vi "Pump Module (Main).vi"(7 "Name of Parent Panel":string="Main.vi", 9 "New Center Coords":T1={"Horizontal"=470, "Vertical"=200}, 10 "Config":variant, 11 "Main UI Message Queue":refnum<queue>) -> ()   [LabVIEW 2018, in "Pump Module.lvlib"]
doc: "This Continuous Measurement sample project is based on the Queued Message Handler template.\n\nThe Event Handling Loop generates messages based on user interface actions.\n\nThe Message Handling Loop processes messages generated by the Event Handling Loop, or by other messages. There are also Acquisition and Logging message handling loop subVIs, and a chart updating loop."
uses:
  Pump Module.lvlib
  support/Message Queue/Message Cluster.ctl
  <vilib>/Utility/miscctls.llb/LVPoint32TypeDef.ctl
  controls/UI Data.ctl
  controls/UI State.ctl
  Pump Module State Cluster.ctl
  Pump Module Config Cluster.ctl
  Pump Module Settings Cluster.ctl
  Measure Instrument/PID 2 Output Enum.ctl
  Ismatec ISM 831C/Controls/Ismatech ISM831C Settings Cluster.ctl
  Ismatec 78001/Ismatec 4083.ctl
  Masterflex 7550-30/Controls/Settings Cluster.ctl
  VICI M50 Party Mode/Settings Cluster.ctl
  Tacmina QI/Tacmina QI DAQ Setting.ctl
  KNF Pump/Settings Cluster plus SIMDOS.ctl
  ASIA Pump/Pump Settings.ctl
  FLOM Pump/Settings Cluster.ctl
  SSI PR Class/SSI PR or LD Settings Cluster.ctl
  Masterflex 75211/Masterflex 75211 DAQ Setting.ctl
  Measure Instrument/State Enum.ctl
  Sequencing/Squence Update Cluster.ctl
  Pump Module Display.ctl
  support/Message Queue/Enqueue Message (Single).vi
  support/User Event - Stop/User Event - Stop.lvlib
  support/Support Library.lvlib
  support/Message Queue/Message Queue.lvlib
  Measure Instrument/Pump Module Engine.lvlib
  Masterflex 7550-30/Masterflex 7550-30.lvlib
  Ismatec ISM 831C/Ismatec ISM 831C.lvlib
  Measure Instrument/Feed Module Engine.lvlib
  Tacmina QI/Tacmina QI.lvlib
  KNF Pump/KNF SIMDOS.lvlib
  ASIA Pump.lvlib
  Sequencing/Sequencing Library.lvlib
  VICI M50 Party Mode/VICI M6 M50 Party Mode.lvlib
  Pump Settings Dialog.vi
  FLOM Pump/FLOM Pump.lvlib
  support/Command Log VIs/Command Logging.lvlib
  SSI PR Class/SSI PR or LD Pump.lvlib
  Masterflex 75211/Masterflex 75211.lvlib
  Ismatec 78001/Ismatec 4308.lvlib
  Report Generation/Report Generation.lvlib
panel:
  out "Calibration Enum":dbl
  in  "Settings Button":bool
  out "Original Width":u32
  out "Original Height":u32
  out "H/W":dbl
  out "Sequence Started":bool
  out "ScanCode":i16
  out "Log File path":path
  out "Status":string
  in  "Exit":bool
  out "Display Cluster":T2 {"Total ml" format="%#.1g"; "ml/min" format="%#_5g"; "PSIG" format="%#_5g"; "Pump %" format="%#_5g"}
  out "Ring":u16(ring)=2
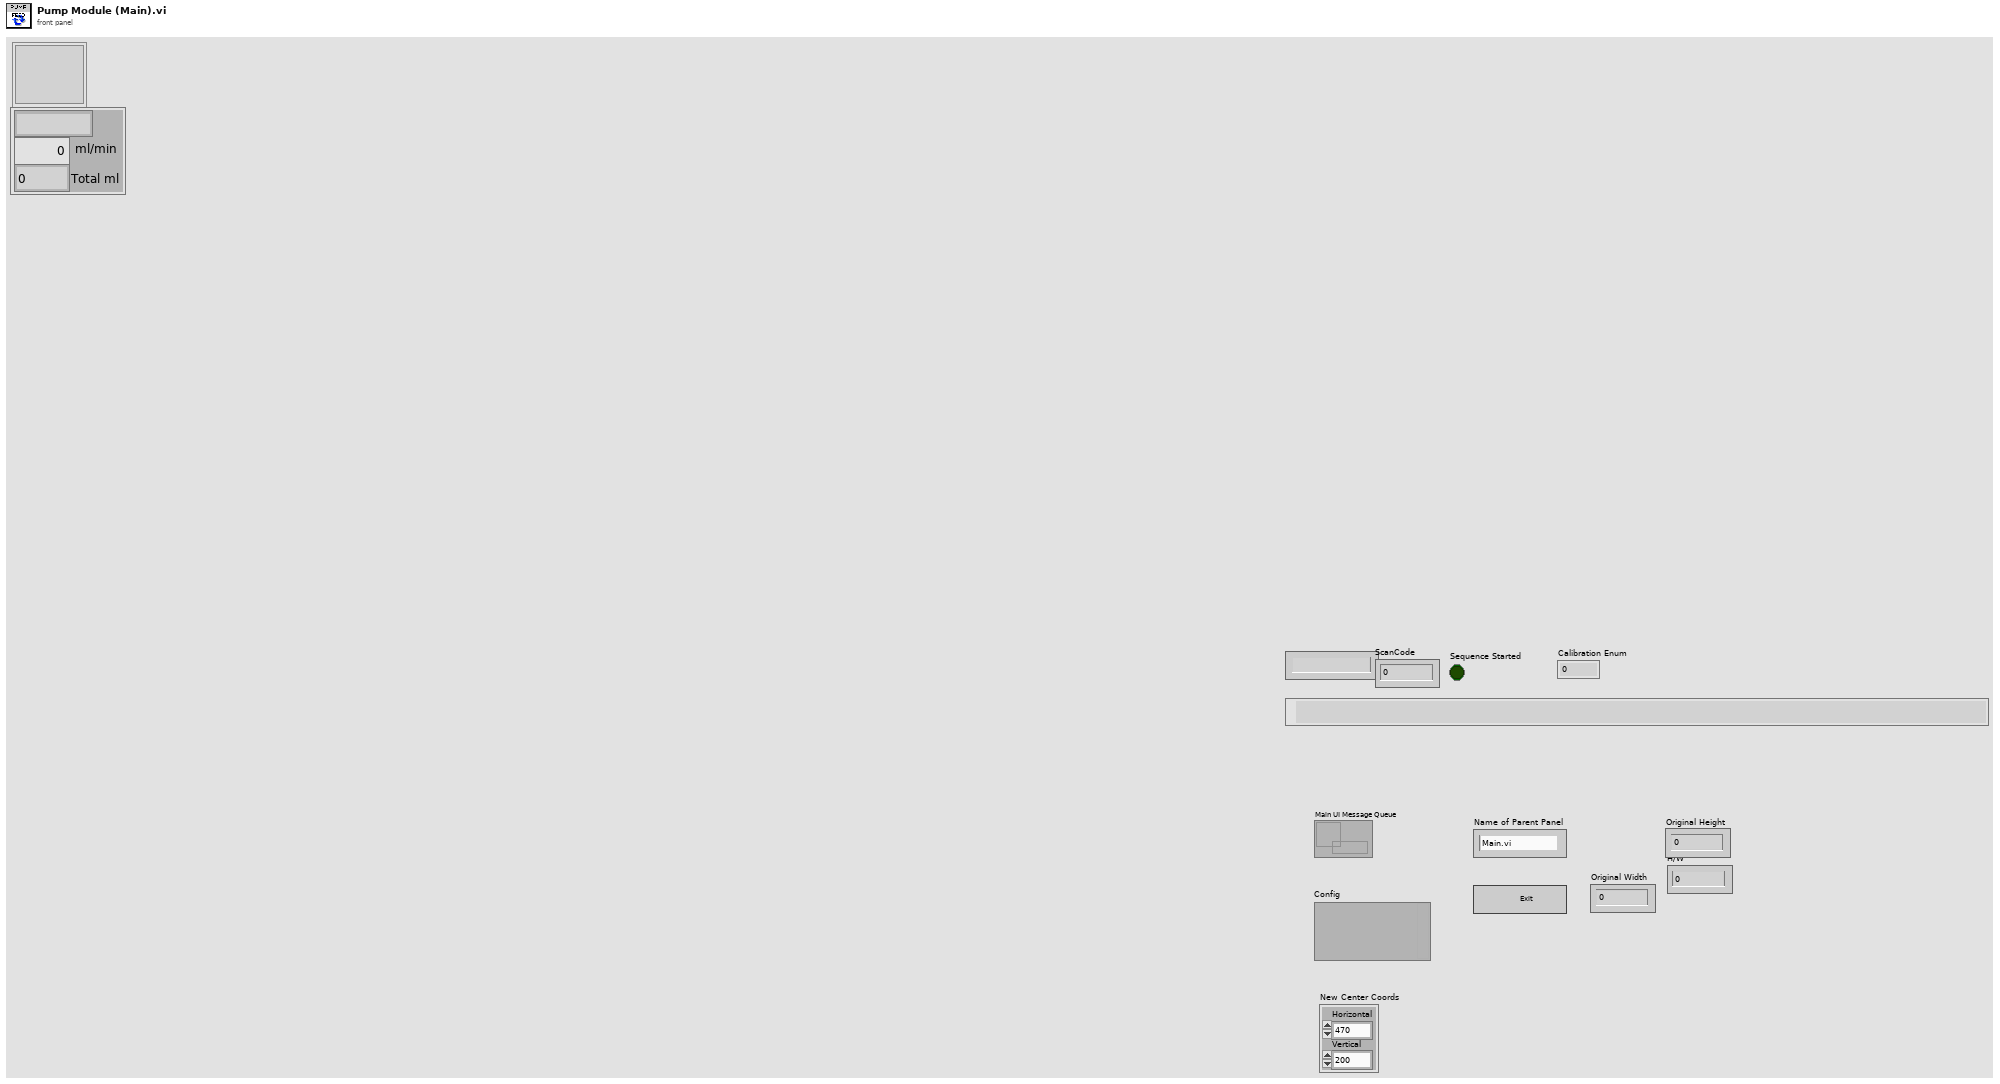
[diagram p1: front panel]
types:
  T1 = typedef "LVPoint32TypeDef.ctl" = cluster{"Horizontal":i32, "Vertical":i32}
  T2 = cluster{"User Name":string, "Pump %":dbl, "PSIG":dbl, "ml/min":dbl, "Total ml":dbl}
  T3 = typedef "Pump Module.lvlib/Pump Module Config Cluster.ctl" = cluster{"GUID":string, "Drop Coords":T1, "Process Name":string, "User name":string, "Queue Name":string, "Settings":T4, "Load Count":i32}
  T4 = typedef "Pump Module.lvlib/Pump Module Settings Cluster.ctl" = cluster{"Cycle Period":dbl, "Manual Entry":dbl, "Output Device":T5, "Ismatech":T6, "Ismatech 3 Channel Settings":T7, "Masterflex":T8, "VICI Settings":T9, "Tacmina Settings":T10, "KNF SIMDOS Settings":T11, "ASIA Pump C":T12, "FLOM Settings":T13, "SSI PR/LD Settings":T14, "SSI P40 Settings":T14, "Masterflex 75211 Settings":T15, "Pump Calibration File":path, "Calibration Slope":dbl, "Calibration Y Intercept":dbl, "Pump Cal Enum":u16, "Reset Totalizer":bool}
  T5 = typedef "PID 2 Output Enum.ctl" = enum16{"Default", "Ismatec ISM 4308", "Ismatec ISM 831C", "Masterflex 7550-30", "VICI M6", "VICI M50", "Tacmina QI", "KNF SIMDOS", "ASIA Type C", "FLOM UI-22-11", "SSI PR/LD", "SSI P40", "Masterflex 75211-70"}
  T6 = typedef "Ismatec ISM 831C.lvlib/Ismatech ISM831C Settings Cluster.ctl" = cluster{"VISA resource name":refnum<visa-resource-name>, "Simulated?":bool, "Pump Number":dbl, "Reverse?":bool}
  T7 = typedef "Ismatec 4308.lvlib/Ismatec 4083.ctl" = cluster{"VISA resource name":refnum<visa-resource-name>, "Pump Number":i16, "Channel Number":i16, "Simulated?":bool, "Reverse?":bool}
  T8 = typedef "Masterflex 7550-30.lvlib/Settings Cluster.ctl" = cluster{"VISA resource name":refnum<visa-resource-name>, "Simulated?":bool, "Pump Number":dbl, "Reverse?":bool}
  T9 = typedef "VICI M6 M50 Party Mode.lvlib/Settings Cluster.ctl" = cluster{"VISA resource name":refnum<visa-resource-name>, "Pump ID":string, "Pump Head Vol":dbl, "Reverse?":bool, "Simulated?":bool}
  T10 = typedef "Tacmina QI.lvlib/Tacmina QI DAQ Setting.ctl" = cluster{"Analog DAQ Task":refnum<k21>, "Digital DAQ Task":refnum<k21>}
  T11 = typedef "KNF SIMDOS.lvlib/Settings Cluster plus SIMDOS.ctl" = cluster{"VISA resource name":refnum<visa-resource-name>, "Simulated?":bool}
  T12 = typedef "ASIA Pump.lvlib/Pump Settings.ctl" = cluster{"ASIA Pump #":i32, "channel":i32, "Simulated":bool}
  T13 = typedef "FLOM Pump.lvlib/Settings Cluster.ctl" = cluster{"VISA resource name":refnum<visa-resource-name>, "Simulated?":bool, "Pump Number":dbl}
  T14 = typedef "SSI PR or LD Pump.lvlib/SSI PR or LD Settings Cluster.ctl" = cluster{"VISA resource name":refnum<visa-resource-name>, "Simulated?":bool}
  T15 = typedef "Masterflex 75211.lvlib/Masterflex 75211 DAQ Setting.ctl" = cluster{"Analog DAQ Task":refnum<k21>, "Digital DAQ Task":refnum<k21>}
  T16 = enum32{"Invalid", "Default", "Floating", "Floating/Auto-Hide", "Modal"}
  T17 = typedef "UI State.ctl" = enum16{"Idle", "Acquiring and Logging", "Waiting for Exit", "Waiting for Exit (Acq Stopped)", "Waiting for Exit (Log Stopped)", "Waiting for Stop", "Waiting for Stop (Acq Stopped)", "Waiting for Stop (Log Stopped)"}
  T18 = typedef "UI Data.ctl" = cluster{"Start Ref":refnum<vi>, "Trigger Ref":refnum<vi>, "Stop Ref":refnum<vi>, "Settings Ref":refnum<vi>, "Status Ref":refnum<vi>, "Exit Ref":refnum<vi>, "Data Ref":refnum<vi>}
  T19 = typedef "Pump Module.lvlib/Pump Module State Cluster.ctl" = cluster{"Pump Module Config":T3, "State":T20, "Start Time":timestamp, "Current Time":timestamp, "First Iteration":bool, "Data":cluster{"Pump Speed":dbl, "Totalized":dbl}, "Process Name":string, "Pump On?":bool}
  T20 = typedef "Feed Module.lvlib/Feed Module Engine.lvlib/State Enum.ctl" = enum16{"Measuring", "Idle", "Paused"}
  T21 = typedef "LVPointTypeDef.ctl" = cluster{"Horizontal":i16, "Vertical":i16}
  T22 = typedef "Pump Module.lvlib/All Message Queues.ctl" = cluster{"Engine":refnum<queue>, "Pump UI":refnum<queue>, "Pump Engine":refnum<queue>, "Pump Display":refnum<queue>}
  T23 = typedef "Pump Module.lvlib/Pump Module Display.ctl" = cluster{"Pump On?":enum16{"Off", "On", "Not Initialized"}, "Cycle Period":dbl, "Current Pump Speed":dbl, "Current Pump Pressure":dbl, "Current Pump Flow":dbl, "Totalized":dbl, "Output":T5}
  T24 = typedef "LVRectTypeDef.ctl" = cluster{"Left":i16, "Top":i16, "Right":i16, "Bottom":i16}
  T25 = cluster{"Shift":bool, "Ctrl":bool, "Alt":bool, "Cmd":bool, "Opt":bool}
  T26 = typedef "Sequencing Library.lvlib/Squence Update Cluster.ctl" = cluster{"Auto?":bool, "Manual Entry":dbl, "Setpoint":dbl}
  T27 = enum8{"Enabled", "Disabled", "Disabled and Grayed Out"}
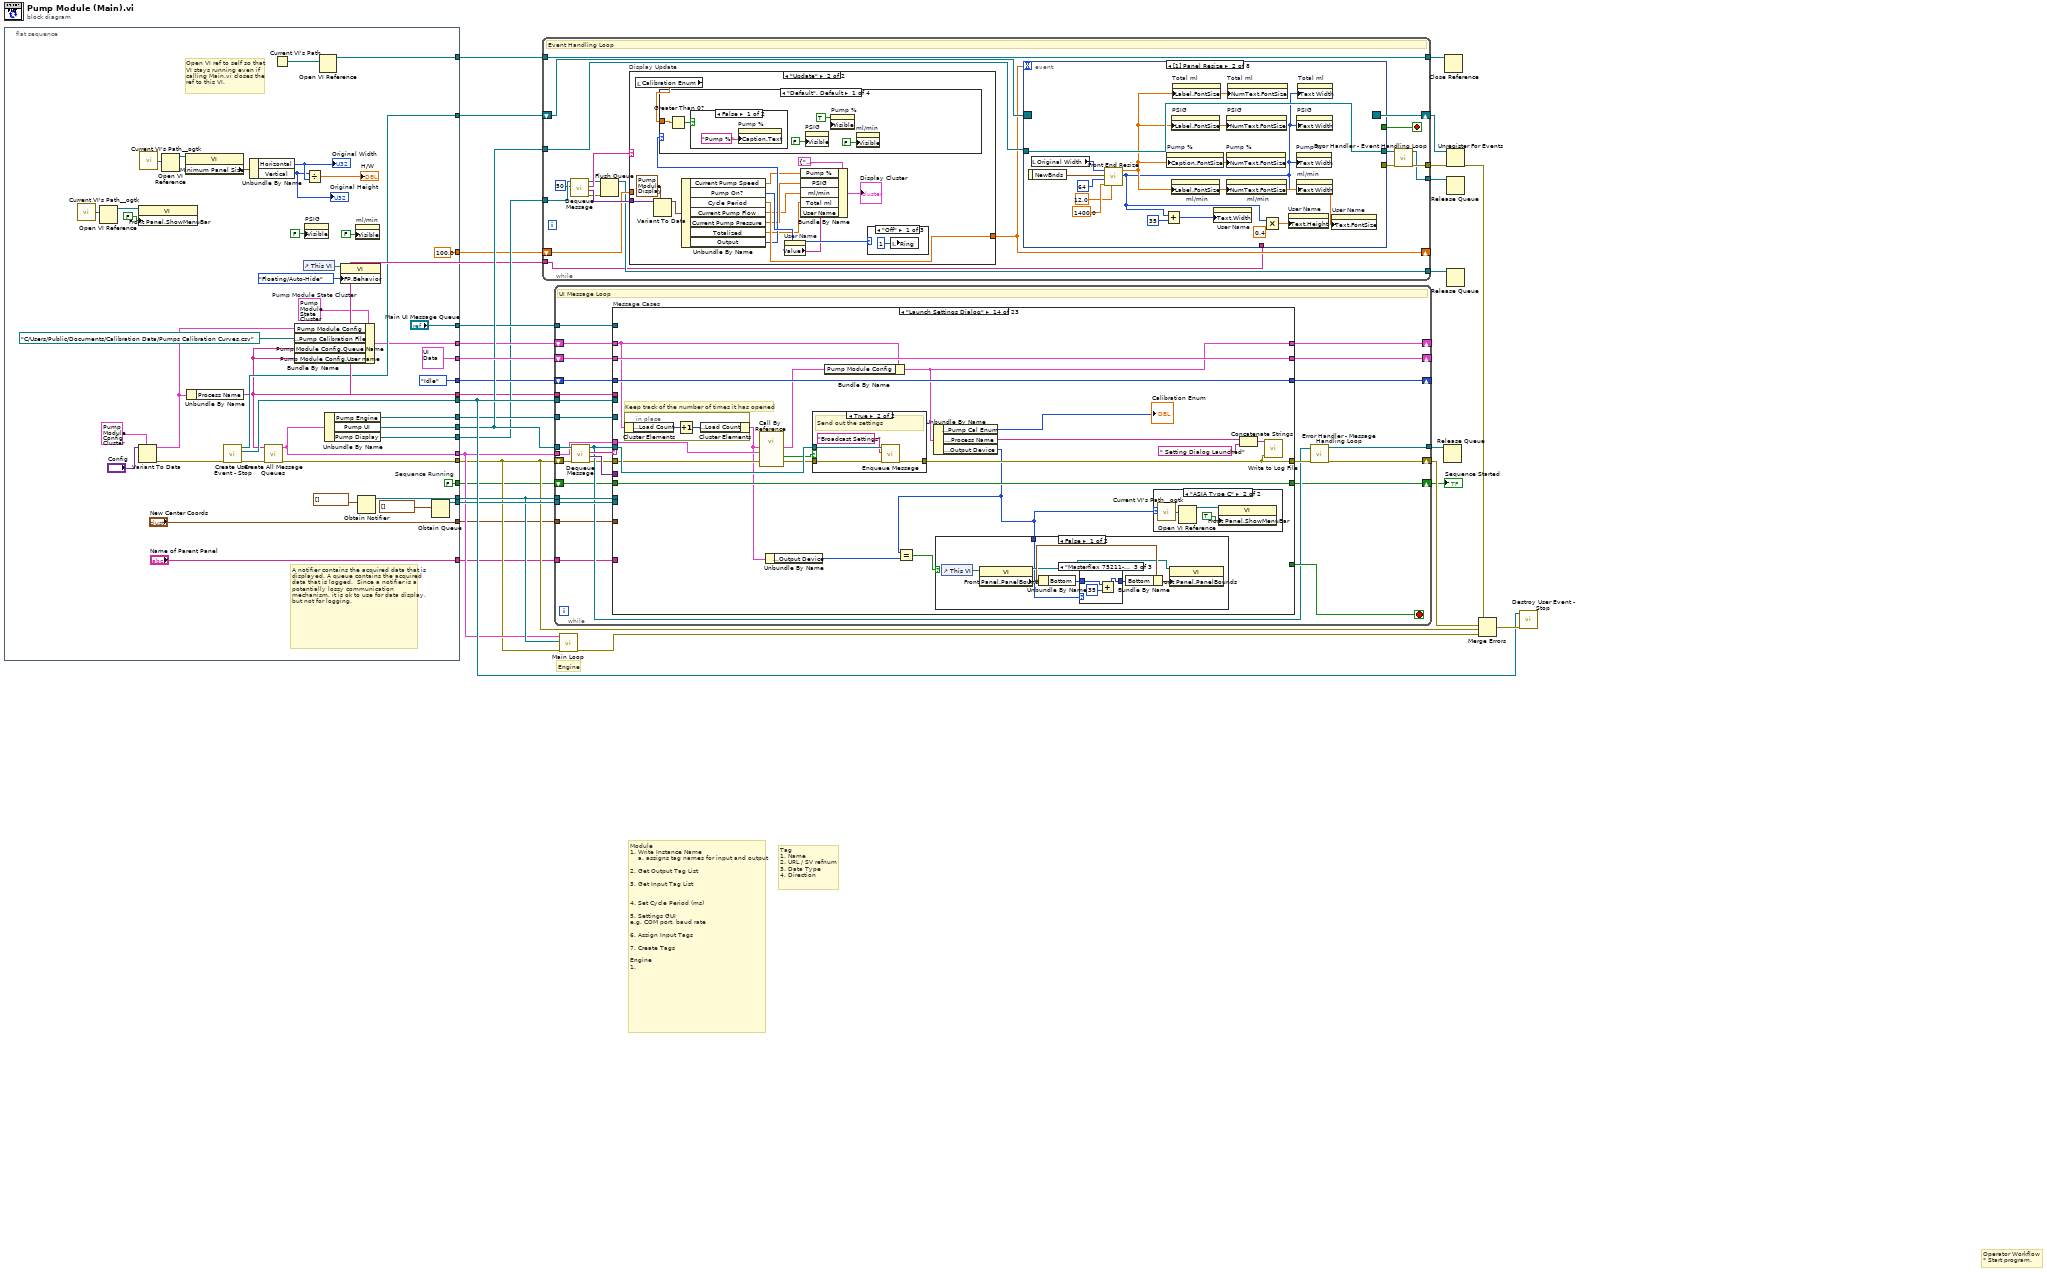
[diagram p0: block diagram]
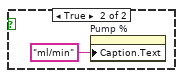
[diagram p3: hidden frame]
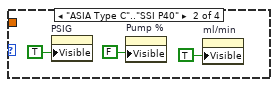
[diagram p4: hidden frame]
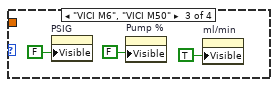
[diagram p5: hidden frame]
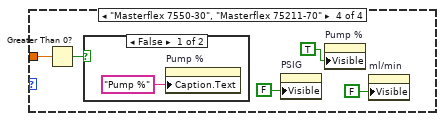
[diagram p6: hidden frame]
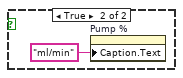
[diagram p7: hidden frame]
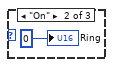
[diagram p8: hidden frame]
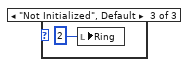
[diagram p9: hidden frame]
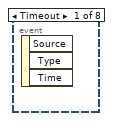
[diagram p10: hidden frame]
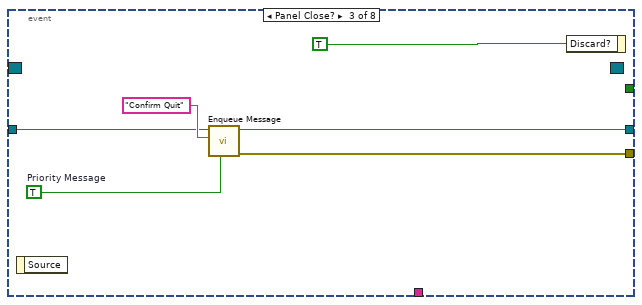
[diagram p11: hidden frame]
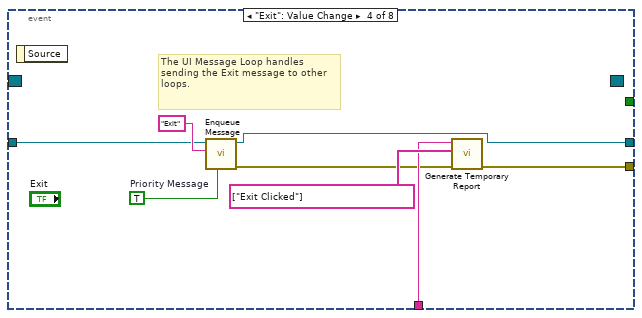
[diagram p12: hidden frame]
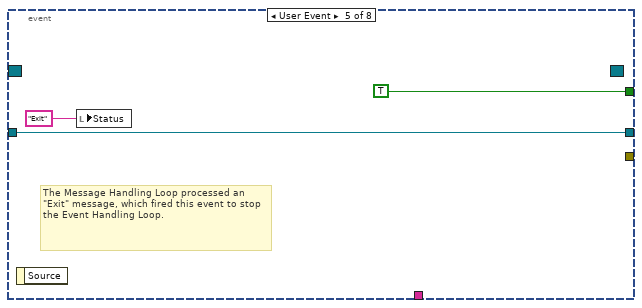
[diagram p13: hidden frame]
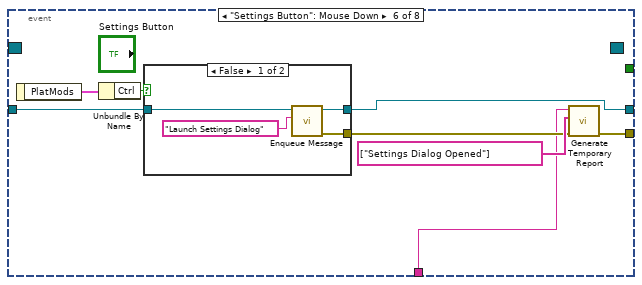
[diagram p14: hidden frame]
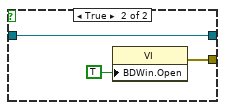
[diagram p15: hidden frame]
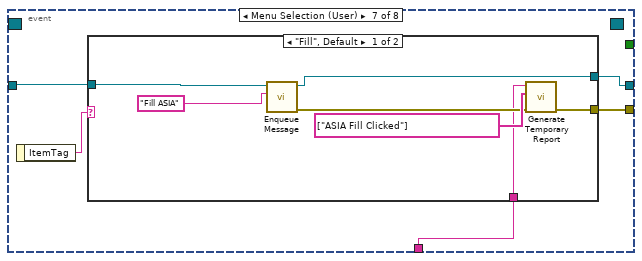
[diagram p16: hidden frame]
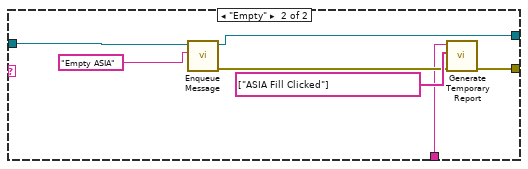
[diagram p17: hidden frame]
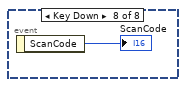
[diagram p18: hidden frame]
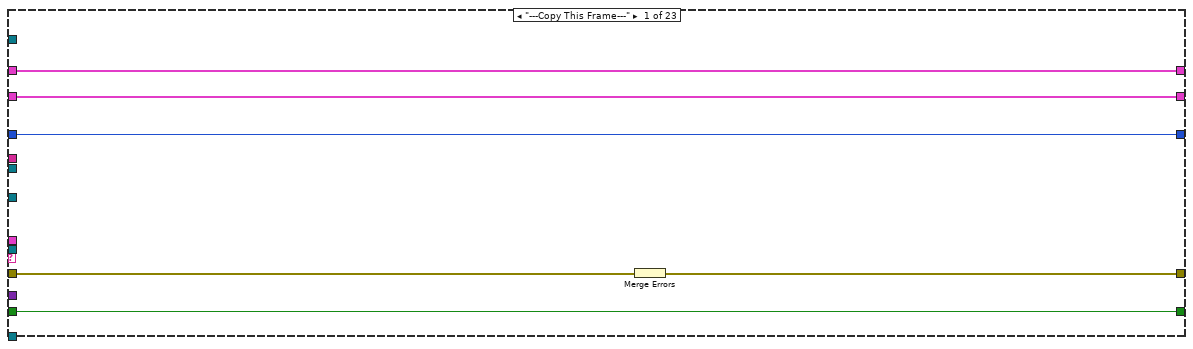
[diagram p19: hidden frame]
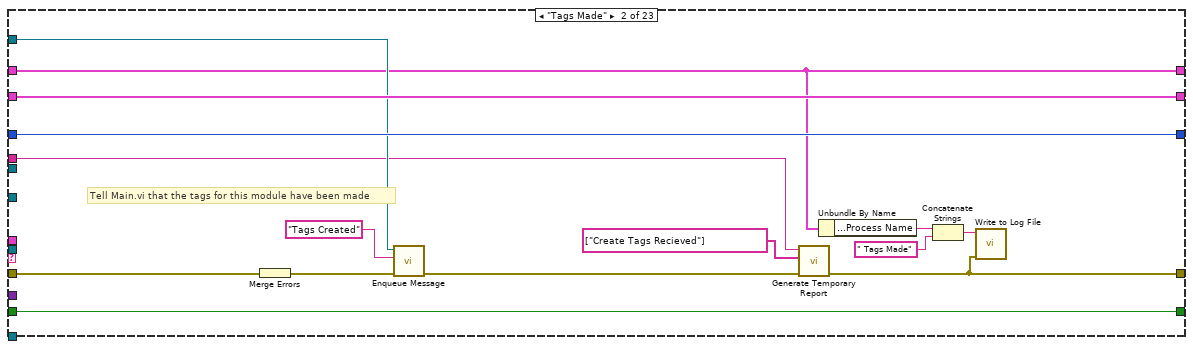
[diagram p20: hidden frame]
diagram:
  # "Engine"
  # "Operator Workflow\n* Start program."
  # "Module \n1. Write Instance Name\n    a. assigns tag names for input and output\n\n2. Get Output Tag List\n\n3. Get Input Tag List\n\n\n4. Set Cycle Period (ms)\n\n5. Settings GUI\ne.g. COM port, baud rate\n\n6. Assign Input Tags\n\n7. Create Tags\n\nEngine\n1."
  # "Tag\n1. Name\n2. URL / SV refnum\n3. Data Type\n4. Direction"
  n1 = flat-sequence {
    tunnel: [w72] -> w27
    tunnel: [w71] -> w26
    tunnel: [T18 {"Start Ref"=refnum, "Trigger Ref"=refnum, "Stop Ref"=refnum, "Settings Ref"=refnum, "Status Ref"=refnum, "Exit Ref"=refnum, "Data Ref"=refnum} ("Measurement UI Controls")] -> w23
    tunnel: [w69] -> w22
    tunnel: [UI_State."Idle" ("UI State")] -> w21
    tunnel: [w65] -> w20
    tunnel: [w64] -> w19
    tunnel: [w63] -> w17
    tunnel: [w62] -> w15
    tunnel: [w60] -> w14
    tunnel: ["Main UI Message Queue"] -> w13
    tunnel: [w55] -> w12
    tunnel: [w53] -> w11
    tunnel: [w52] -> w10
    tunnel: ["New Center Coords"] -> w9
    tunnel: ["Name of Parent Panel"] -> w8
    tunnel: [w49] -> w6
    tunnel: [100.0 ("Cycle Period")] -> w5
    tunnel: [w42] -> w1
    frame #0 {
      w49 = FALSE  # Sequence Running
      w56 = T19 {"Pump Module Config"={"GUID"="", "Drop Coords"={"Horizontal"=0, "Vertical"=0}, "Process Name"="", "User name"="", "Queue Name"="", "Settings"={"Cycle Period"=500.0, "Manual Entry"=0.0, "Output Device"=enum."VICI M6", "Ismatech"={"VISA resource name"="", "Simulated?"=TRUE, "Pump Number"=1.0, "Reverse?"=FALSE}, "Ismatech 3 Channel Settings"={"VISA resource name"="", "Pump Number"=1, "Channel Number"=0, "Simulated?"=TRUE, "Reverse?"=FALSE}, "Masterflex"={"VISA resource name"="", "Simulated?"=TRUE, "Pump Number"=1.0, "Reverse?"=FALSE}, "VICI Settings"={"VISA resource name"="", "Pump ID"="", "Pump Head Vol"=0.0, "Reverse?"=FALSE, "Simulated?"=TRUE}, "Tacmina Settings"={"Analog DAQ Task"="", "Digital DAQ Task"=""}, "KNF SIMDOS Settings"={"VISA resource name"="", "Simulated?"=TRUE}, "ASIA Pump C"={"ASIA Pump #"=0, "channel"=0, "Simulated"=FALSE}, "FLOM Settings"={"VISA resource name"="", "Simulated?"=TRUE, "Pump Number"=0.0}, "SSI PR/LD Settings"={"VISA resource name"="", "Simulated?"=FALSE}, "SSI P40 Settings"={"VISA resource name"="", "Simulated?"=FALSE}, "Masterflex 75211 Settings"={"Analog DAQ Task"="", "Digital DAQ Task"=""}, "Pump Calibration File"=path "", "Calibration Slope"=0.0, "Calibration Y Intercept"=0.0, "Pump Cal Enum"=0, "Reset Totalizer"=FALSE}, "Load Count"=0}, "State"=enum."Idle", "Start Time"=timestamp(0 s since 1904-01-01), "Current Time"=timestamp(0 s since 1904-01-01), "First Iteration"=FALSE, "Data"={"Pump Speed"=0.0, "Totalized"=0.0}, "Process Name"="", "Pump On?"=FALSE}  # Pump Module State Cluster
      # "Open VI ref to self so that\nVI stays running even if\ncalling Main.vi closes the\nref to this VI."
      # "A notifier contains the acquired data that is displayed. A queue contains the acquired data that is logged.  Since a notifier is a potentially lossy communication mechanism, it is ok to use for data display, but not for logging."
      n2 = call <userlib>:"Current VI's Path__ogtk.vi"() -> ("Current VI's Path (+ Relative)"=w33:path)  [unwired: 1 in]
      n3 = Open VI Reference(vi path=w33) -> (vi reference=w31:refnum<vi>)  [unwired: 5 in, 1 out]
      n4 = property class="VI"(reference=w31, "Front Panel.ShowMenuBar"=FALSE ("Front Panel Window:Show Menu Bar")) -> ()  [unwired: 1 in, 2 out]
      n5 = Variant To Data(type=T3 {"GUID"="", "Drop Coords"={"Horizontal"=0, "Vertical"=0}, "Process Name"="", "User name"="", "Queue Name"="", "Settings"={"Cycle Period"=500.0, "Manual Entry"=0.0, "Output Device"=enum."VICI M6", "Ismatech"={"VISA resource name"="", "Simulated?"=TRUE, "Pump Number"=1.0, "Reverse?"=FALSE}, "Ismatech 3 Channel Settings"={"VISA resource name"="", "Pump Number"=1, "Channel Number"=0, "Simulated?"=TRUE, "Reverse?"=FALSE}, "Masterflex"={"VISA resource name"="", "Simulated?"=TRUE, "Pump Number"=1.0, "Reverse?"=FALSE}, "VICI Settings"={"VISA resource name"="", "Pump ID"="", "Pump Head Vol"=0.0, "Reverse?"=FALSE, "Simulated?"=TRUE}, "Tacmina Settings"={"Analog DAQ Task"="", "Digital DAQ Task"=""}, "KNF SIMDOS Settings"={"VISA resource name"="", "Simulated?"=TRUE}, "ASIA Pump C"={"ASIA Pump #"=0, "channel"=0, "Simulated"=FALSE}, "FLOM Settings"={"VISA resource name"="", "Simulated?"=TRUE, "Pump Number"=0.0}, "SSI PR/LD Settings"={"VISA resource name"="", "Simulated?"=FALSE}, "SSI P40 Settings"={"VISA resource name"="", "Simulated?"=FALSE}, "Masterflex 75211 Settings"={"Analog DAQ Task"="", "Digital DAQ Task"=""}, "Pump Calibration File"=path "", "Calibration Slope"=0.0, "Calibration Y Intercept"=0.0, "Pump Cal Enum"=0, "Reset Totalizer"=FALSE}, "Load Count"=0} ("Feed Module Config"), Variant="Config") -> (data=w58:T3, error out=w59:errorcluster)  [unwired: 1 in]
      n6 = call <userlib>:"Current VI's Path__ogtk.vi"() -> ("Current VI's Path (+ Relative)"=w38:path)  [unwired: 1 in]
      n7 = Open VI Reference(vi path=w38) -> (vi reference=w37:refnum<vi>)  [unwired: 5 in, 1 out]
      n8 = property class="VI"(reference=w37) -> ("Minimum Panel Size"=w36:T21)  [unwired: 1 in, 2 out]
      n9 = Unbundle By Name(w58) -> ("Process Name"=w42:string)
      n10 = call "Create User Event - Stop.vi"("error in (no error)"=w59) -> ("error out"=w54:errorcluster, "User Event - Stop"=w71:refnum<user-event>, "Stop Event Registration Refnum"=w72:refnum<event-registration>)  [unwired: 8 in]
      n11 = Unbundle By Name(w36) -> ("Horizontal"=w35:i16, "Vertical"=w34:i16)
      "Original Width" <- w35
      "Original Height" <- w34
      n12 = call "Create All Message Queues.vi"("error in (no error)"=w54, "Process Name"=w42) -> ("error out"=w52:errorcluster, "Message Queues"=w53:T22)  [unwired: 8 in]
      n13 = Current VI's Path() -> (path=w61:path)
      n14 = Bundle By Name(cluster=w56, "Pump Module Config"=w58, "Pump Module Config.Settings.Pump Calibration File"=path "C:/Users/Public/Documents/Calibration Data/Pumps Calibration Curves.csv", "Pump Module Config.Queue Name"=w42, "Pump Module Config.User name"=w42) -> (w60:T19)
      n15 = control-ref of="This VI"() -> (w44:refnum<vi>)
      n16 = property on="PSIG" class="DigNum (strict)"("Visible"=FALSE) -> ()  [unwired: 2 in, 2 out]
      n17 = Divide(x=w34, y=w35) -> (x/y=→"H/W":dbl)
      n18 = Open VI Reference(vi path=w61) -> (vi reference=w62:refnum<vi>)  [unwired: 5 in, 1 out]
      n19 = Unbundle By Name(w53) -> ("Pump Engine"=w65:refnum<queue>, "Pump UI"=w69:refnum<queue>, "Pump Display"=w55:refnum<queue>)
      n20 = property class="VI"(reference=w44, "FP.Behavior"=T16."Floating/Auto-Hide" ("Front Panel Window:Behavior")) -> ()  [unwired: 1 in, 2 out]
      n21 = property on="ml/min" class="DigNum (strict)"("Visible"=FALSE) -> ()  [unwired: 2 in, 2 out]
      n22 = Obtain Notifier(notification data type=waveform(dbl)[] []) -> (notifier out=w63:refnum<notifier>)  [unwired: 3 in, 2 out]
      n23 = Obtain Queue(element data type=waveform(dbl)[] []) -> (queue out=w64:refnum<queue>)  [unwired: 4 in, 2 out]
    }
  }
  n24 = while {
    tunnel: w22 -> [w85]
    tunnel: [w87] -> w29
    shift-right: [w86] -> w24
    shift-left: w27 -> [w91]
    tunnel: [w84] -> w16
    tunnel: w15 -> [w84]
    tunnel: w12 -> [w83]
    shift-right: [w80] -> _
    shift-left: w5 -> [w79]
    tunnel: [w75] -> w4
    tunnel: [w74] -> w3
    tunnel: w1 -> [w73]
    stop <- w90 stop-if-true
    # "Event Handling Loop"
    n25 = call "Dequeue Message.vi"("timeout in ms (-1)"=50, "Message Queue"=w83) -> ("error out"=w76:errorcluster, "Message Data"=w81:variant, "Message"=w82:string, "dup Message Queue"=w77:refnum<queue>)  [unwired: 6 in]
    n26 = Flush Queue(queue=w77, error in (no error)=w76) -> (queue out=w74:refnum<queue>)  [unwired: 2 out]
    n27 = case "Display Update" shown="\"Update\"" w82 {
      tunnel: w81 -> [_ w106]
      tunnel: [w92 w103] -> w80
      tunnel: w79 -> [w92 _]
      frame "False", Default {
      }
      frame "Update" {
        n28 = local read "Calibration Enum"() -> (w95:dbl)
        n29 = Variant To Data(type=T23 {"Pump On?"=enum."Off", "Cycle Period"=500.0, "Current Pump Speed"=0.0, "Current Pump Pressure"=0.0, "Current Pump Flow"=0.0, "Totalized"=0.0, "Output"=enum."Default"} ("FM Display"), Variant=w106) -> (data=w105:T23)  [unwired: 1 in, 1 out]
        n30 = Unbundle By Name(w105) -> ("Current Pump Speed"=w99:dbl, "Pump On?"=w104:enum16{"Off", "On", "Not Initialized"}, "Cycle Period"=w103:dbl, "Current Pump Flow"=w98:dbl, "Current Pump Pressure"=w100:dbl, "Totalized"=w96:dbl, "Output"=w101:T5)
        n31 = case shown="\"Default\", Default" w101 {
          tunnel: w95 -> [w107 _ _ w120]
          frame "Default", Default {
            n32 = Greater Than 0?(x=w107) -> (x > 0?=w108:bool)
            n33 = case shown="False" w108 {
              frame False {
                n34 = property on="Pump %" class="DigNum (strict)"("Caption.Text"="Pump %" ("Label.Text")) -> ()  [unwired: 2 in, 2 out]
              }
              frame True {
                n35 = property on="Pump %" class="DigNum (strict)"("Caption.Text"="ml/min" ("Label.Text")) -> ()  [unwired: 2 in, 2 out]
              }
            }
            n36 = property on="PSIG" class="DigNum (strict)"("Visible"=FALSE) -> ()  [unwired: 2 in, 2 out]
            n37 = property on="Pump %" class="DigNum (strict)"("Visible"=TRUE) -> ()  [unwired: 2 in, 2 out]
            n38 = property on="ml/min" class="DigNum (strict)"("Visible"=FALSE) -> ()  [unwired: 2 in, 2 out]
          }
          frame "ASIA Type C".."SSI P40" {
            n39 = property on="PSIG" class="DigNum (strict)"("Visible"=TRUE) -> ()  [unwired: 2 in, 2 out]
            n40 = property on="Pump %" class="DigNum (strict)"("Visible"=FALSE) -> ()  [unwired: 2 in, 2 out]
            n41 = property on="ml/min" class="DigNum (strict)"("Visible"=TRUE) -> ()  [unwired: 2 in, 2 out]
          }
          frame "VICI M6", "VICI M50" {
            n42 = property on="PSIG" class="DigNum (strict)"("Visible"=FALSE) -> ()  [unwired: 2 in, 2 out]
            n43 = property on="Pump %" class="DigNum (strict)"("Visible"=FALSE) -> ()  [unwired: 2 in, 2 out]
            n44 = property on="ml/min" class="DigNum (strict)"("Visible"=TRUE) -> ()  [unwired: 2 in, 2 out]
          }
          frame "Masterflex 7550-30", "Masterflex 75211-70" {
            n45 = Greater Than 0?(x=w120) -> (x > 0?=w121:bool)
            n46 = case shown="False" w121 {
              frame False {
                n47 = property on="Pump %" class="DigNum (strict)"("Caption.Text"="Pump %" ("Label.Text")) -> ()  [unwired: 2 in, 2 out]
              }
              frame True {
                n48 = property on="Pump %" class="DigNum (strict)"("Caption.Text"="ml/min" ("Label.Text")) -> ()  [unwired: 2 in, 2 out]
              }
            }
            n49 = property on="PSIG" class="DigNum (strict)"("Visible"=FALSE) -> ()  [unwired: 2 in, 2 out]
            n50 = property on="Pump %" class="DigNum (strict)"("Visible"=TRUE) -> ()  [unwired: 2 in, 2 out]
            n51 = property on="ml/min" class="DigNum (strict)"("Visible"=FALSE) -> ()  [unwired: 2 in, 2 out]
          }
        }
        n52 = property on="User Name" class="Str"() -> ("Value"=w93:string)  [unwired: 2 in, 2 out]
        n53 = Bundle By Name(cluster=T2 {"User Name"="", "Pump %"=0.0, "PSIG"=0.0, "ml/min"=0.0, "Total ml"=0.0} ("Display Cluster"), "Pump %"=w99, "PSIG"=w100, "ml/min"=w98, "Total ml"=w96, "User Name"=w93) -> (→"Display Cluster":T2)
        n54 = case shown="\"Off\"" w104 {
          frame "Off" {
            n55 = local write "Ring"(u16 1 ("Ring")) -> ()
          }
          frame "On" {
            "Ring" <- u16 0 ("Ring")
          }
          frame "Not Initialized", Default {
            n56 = local write "Ring"(u16 2 ("Ring")) -> ()
          }
        }
      }
    }
    n57 = event shown="[1] Panel Resize" {
      selector: w91 -> [_ _ _ _ _ _ _ _]
      dyn-events: [_ _ _ _ _ _ _ _] -> w86
      timeout: w80 -> [_ _ _ _ _ _ _ _]
      tunnel: [_ _ _ _ TRUE ("Discard?") _ _ _] -> w90
      tunnel: w85 -> [_ w141 w144 w153 w156 w165 w178 _]
      tunnel: [_ _ w142 w148 _ w160 w176 _] -> w88
      tunnel: [_ w141 w143 w152 w156 w166 w175 _] -> w89
      tunnel: w73 -> [_ _ _ w150 _ w159 w174 _]
      event Timeout {
        n58 = event-data() -> ()  [unwired: 1 in, 3 out]
      }
      event Panel Resize {
        n59 = event-data() -> ("NewBnds"=w136:T24)  [unwired: 1 in]
        n60 = local read "Original Width"() -> (w137:u32)
        n61 = call "Front End Resize.vi"("Starting Font"=12.0, "Area to Font Division"=1400.0, "Original Text Box Width"=64, "NewBnds"=w136, "Original Panel Width"=w137) -> ("New Text Box Width"=w130:u64, "New Font Size"=w135:dbl)  [unwired: 5 in]
        n62 = Add(x=w130, y=u64 35) -> (x+y=w131:u64)
        n63 = property on="Pump %" class="DigNum (strict)"("Caption.FontSize"=w135) -> ()  [unwired: 2 in, 2 out]
        n64 = property on="PSIG" class="DigNum (strict)"("Label.FontSize"=w135) -> ()  [unwired: 2 in, 2 out]
        n65 = property on="ml/min" class="DigNum (strict)"("Label.FontSize"=w135) -> ()  [unwired: 2 in, 2 out]
        n66 = property on="Total ml" class="DigNum (strict)"("Label.FontSize"=w135) -> ()  [unwired: 2 in, 2 out]
        n67 = property on="User Name" class="Str"("Text.Width"=w131) -> ()  [unwired: 2 in, 2 out]
        n68 = property on="Pump %" class="DigNum (strict)"("NumText.FontSize"=w135) -> ()  [unwired: 2 in, 2 out]
        n69 = property on="PSIG" class="DigNum (strict)"("NumText.FontSize"=w135) -> ()  [unwired: 2 in, 2 out]
        n70 = property on="ml/min" class="DigNum (strict)"("NumText.FontSize"=w135) -> ()  [unwired: 2 in, 2 out]
        n71 = property on="Total ml" class="DigNum (strict)"("NumText.FontSize"=w135) -> ()  [unwired: 2 in, 2 out]
        n72 = Multiply(x=w130, y=0.4) -> (x*y=w134:dbl)
        n73 = property on="User Name" class="Str"("Text.Height"=w134) -> ()  [unwired: 2 in, 2 out]
        n74 = property on="Pump %" class="DigNum (strict)"("Text Width"=w130) -> ()  [unwired: 2 in, 2 out]
        n75 = property on="PSIG" class="DigNum (strict)"("Text Width"=w130) -> ()  [unwired: 2 in, 2 out]
        n76 = property on="ml/min" class="DigNum (strict)"("Text Width"=w130) -> ()  [unwired: 2 in, 2 out]
        n77 = property on="Total ml" class="DigNum (strict)"("Text Width"=w130) -> ()  [unwired: 2 in, 2 out]
        n78 = property on="User Name" class="Str"("Text.FontSize"=w135) -> ()  [unwired: 2 in, 2 out]
      }
      event Panel Close? {
        w145 = TRUE  # Priority Message
        n79 = event-data() -> ()  [unwired: 1 in, 1 out]
        n80 = call-poly "Enqueue Message.vi"("Priority Message? (F)"=w145, "Message"="Confirm Quit", "Message Queue"=w144) -> ("error out"=w142:errorcluster, "dup Message Queue"=w143:refnum<queue>)  [unwired: 7 in]
        n81 = event-data("Discard?"=TRUE) -> ()  [unwired: 1 in, 1 out]
      }
      event "Exit": Value Change {
        w154 = TRUE  # Priority Message
        # "The UI Message Loop handles sending the Exit message to other loops."
        n82 = event-data() -> ()  [unwired: 1 in, 1 out]
        n83 = call-poly "Enqueue Message.vi"("Priority Message? (F)"=w154, "Message"="Exit", "Message Queue"=w153) -> ("error out"=w149:errorcluster, "dup Message Queue"=w152:refnum<queue>)  [unwired: 7 in]
        n84 = call "Generate Temporary Report.vi"("error in (no error)"=w149, "Line of Events"=string[] ["Exit Clicked"], "Module Name"=w150) -> ("error out"=w148:errorcluster)  [unwired: 8 in]
      }
      event User Event {
        # "The Message Handling Loop processed an \"Exit\" message, which fired this event to stop the Event Handling Loop."
        n85 = event-data() -> ()  [unwired: 1 in, 1 out]
        n86 = local write "Status"("Exit" ("Exit String")) -> ()
      }
      event "Settings Button": Mouse Down {
        n87 = event-data() -> ("PlatMods"=w164:T25)  [unwired: 1 in]
        n88 = Unbundle By Name(w164) -> ("Ctrl"=w163:bool)
        n89 = case shown="False" w163 {
          tunnel: [w170 w171] -> w161
          tunnel: [w169 w172] -> w166
          tunnel: w165 -> [w168 w172]
          frame False {
            n90 = call-poly "Enqueue Message.vi"("Message"="Launch Settings Dialog", "Message Queue"=w168) -> ("error out"=w170:errorcluster, "dup Message Queue"=w169:refnum<queue>)  [unwired: 8 in]
          }
          frame True {
            n91 = property class="VI"("BDWin.Open"=TRUE ("Block Diagram Window:Open")) -> (error out=w171:errorcluster)  [unwired: 2 in, 1 out]
          }
        }
        n92 = call "Generate Temporary Report.vi"("error in (no error)"=w161, "Line of Events"=string[] ["Settings Dialog Opened"], "Module Name"=w159) -> ("error out"=w160:errorcluster)  [unwired: 8 in]
      }
      event Menu Selection (User) {
        n93 = event-data() -> ("ItemTag"=w177:string)  [unwired: 1 in]
        n94 = case shown="\"Fill\", Default" w177 {
          tunnel: w178 -> [w184 w191]
          tunnel: [w182 w189] -> w176
          tunnel: [w180 w187] -> w175
          tunnel: w174 -> [w179 w186]
          frame "Fill", Default {
            n95 = call-poly "Enqueue Message.vi"("Message"="Fill ASIA", "Message Queue"=w184) -> ("error out"=w181:errorcluster, "dup Message Queue"=w180:refnum<queue>)  [unwired: 8 in]
            n96 = call "Generate Temporary Report.vi"("error in (no error)"=w181, "Line of Events"=string[] ["ASIA Fill Clicked"], "Module Name"=w179) -> ("error out"=w182:errorcluster)  [unwired: 8 in]
          }
          frame "Empty" {
            n97 = call-poly "Enqueue Message.vi"("Message"="Empty ASIA", "Message Queue"=w191) -> ("error out"=w188:errorcluster, "dup Message Queue"=w187:refnum<queue>)  [unwired: 8 in]
            n98 = call "Generate Temporary Report.vi"("error in (no error)"=w188, "Line of Events"=string[] ["ASIA Fill Clicked"], "Module Name"=w186) -> ("error out"=w189:errorcluster)  [unwired: 8 in]
          }
        }
      }
      event Key Down {
        n99 = event-data() -> ("ScanCode"=→"ScanCode":i16)  [unwired: 1 in]
      }
    }
    n100 = call "Error Handler - Event Handling Loop.vi"("error in (no error)"=w88, "Message Queue"=w89) -> ("dup error in"=w87:errorcluster, "dup Message Queue"=w75:refnum<queue>)  [unwired: 8 in]
  }
  n101 = while {
    tunnel: w22 -> [w215]
    tunnel: w26 -> [w219]
    shift-right: [w209] -> w30
    shift-left: w10 -> [w218]
    shift-right: [w202] -> _
    shift-left: w14 -> [w195]
    shift-right: [w213] -> _
    shift-left: w23 -> [w214]
    tunnel: w17 -> [w212]
    tunnel: w19 -> [w211]
    shift-right: [w206] -> _
    shift-left: w21 -> [w207]
    tunnel: w20 -> [w205]
    tunnel: w13 -> [w203]
    tunnel: w11 -> [w201]
    tunnel: w1 -> [w200]
    tunnel: w9 -> [w199]
    tunnel: w8 -> [w198]
    shift-right: [w197] -> w7
    shift-left: w6 -> [w196]
    tunnel: [w194] -> w2
    stop <- w220 stop-if-true
    # "UI Message Loop"
    n102 = call "Dequeue Message.vi"("error in (no error)"=w218, "Message Queue"=w215) -> ("error out"=w204:errorcluster, "Message Data"=w216:variant, "Message"=w217:string, "dup Message Queue"=w208:refnum<queue>)  [unwired: 6 in]
    n103 = case "Message Cases" shown="\"Launch Settings Dialog\"" w217 {
      selector: w217 -> [_ _ _ _ _ _ _ _ _ _ _ _ _ _ _ _ _ _ _ _ _ w754 w770]
      tunnel: w208 -> [_ _ w248 _ w324 _ w360 _ w427 w442 w472 _ w510 w534 w572 w608 w647 _ _ w711 _ _ _]
      tunnel: w204 -> [w226 w241 w249 w283 w323 w345 w359 w392 w408 w446 w476 w492 w505 w533 w573 w606 w646 w671 w684 w713 w747 w758 _]
      tunnel: [w225 w227 w244 w275 w319 w343 w357 w393 w399 w431 w448 w492 w493 w524 w567 w595 w634 w666 w686 w702 w748 w757 w769] -> w210
      tunnel: [_ _ _ _ _ _ _ _ _ _ TRUE _ _ _ _ _ _ _ _ _ _ _ _] -> w220
      tunnel: w216 -> [_ _ _ _ w325 w342 _ w395 _ w445 w460 _ _ _ _ _ _ _ _ _ w746 _ _]
      tunnel: w219 -> [_ _ _ _ _ _ _ _ _ _ w475 _ _ _ _ _ _ _ _ _ _ _ _]
      tunnel: w195 -> [w222 w232 w243 w288 w317 w352 w356 w390 w406 w433 w453 w483 w498 w523 w568 w599 w642 w672 w685 w715 w737 w756 w775]
      tunnel: w214 -> [w224 w240 w252 w301 w326 w354 w362 w397 w424 w447 w473 w491 w506 w536 w576 w603 w643 w677 w695 w731 w743 w762 w780]
      tunnel: [w224 w240 w252 w301 w326 w354 w362 w397 w424 w447 w473 w490 w506 w536 w576 w603 w643 w677 w695 w731 w743 w762 w780] -> w213
      tunnel: w212 -> [_ _ _ _ _ _ _ _ _ _ w471 _ _ _ _ _ _ _ _ _ _ _ _]
      tunnel: w211 -> [_ _ _ _ _ _ _ _ _ _ w467 _ _ _ _ _ _ _ _ _ _ _ _]
      tunnel: w207 -> [w223 w239 w251 w300 w327 w353 w361 w391 w413 w437 _ _ _ w535 w575 _ _ _ _ w720 w738 w760 w779]
      tunnel: [w223 w239 w250 w300 w327 w353 w358 w391 w414 w437 UI_State."Idle" ("UI State") UI_State."Idle" ("UI State") UI_State."Idle" ("UI State") w535 w574 UI_State."Acquiring and Logging" ("UI State") UI_State."Acquiring and Logging" ("UI State") UI_State."Acquiring and Logging" ("UI State") UI_State."Acquiring and Logging" ("UI State") w721 w738 w760 w779] -> w206
      tunnel: w205 -> [_ _ _ w292 _ _ _ _ w412 _ w459 _ _ _ _ _ _ w675 w693 w719 _ w759 _]
      tunnel: w203 -> [_ w236 _ w298 _ _ _ _ _ _ w461 _ _ _ _ _ _ _ _ _ _ _ _]
      tunnel: [w222 w232 w243 w288 w316 w352 w356 w390 w403 w433 w453 w483 w498 w525 w568 w598 w633 w672 w685 w706 w737 w756 w775] -> w202
      tunnel: w201 -> [_ _ _ w296 _ _ _ _ _ _ _ _ _ w532 _ _ _ _ _ _ _ _ _]
      tunnel: w200 -> [_ w229 _ _ _ _ _ _ _ _ _ _ w501 _ _ _ _ _ _ _ _ _ _]
      tunnel: w199 -> [_ _ _ _ _ _ _ _ _ _ _ _ w503 _ _ _ _ _ _ _ _ _ _]
      tunnel: w198 -> [_ _ _ _ _ _ _ _ _ _ _ _ w502 _ _ _ _ _ _ _ _ _ _]
      tunnel: [w221 w231 w242 w286 w315 w351 w355 w389 w402 w430 w452 w482 w497 w522 w566 w597 w640 w670 w683 w705 w736 w761 w768] -> w197
      tunnel: w196 -> [w221 w231 w242 w286 w315 w351 w355 w389 w402 w430 w452 w482 w497 w522 w566 w597 w638 w670 w683 w705 w736 w761 w768]
      frame "---Copy This Frame---" {
        # "Duplicate this frame when creating new messages.  Change this comment in the duplicated frame to describe this message."
        n104 = Merge Errors(w226) -> (w225:errorcluster)
      }
      frame "Tags Made" {
        # "Tell Main.vi that the tags for this module have been made"
        # "Duplicate this frame when creating new messages.  Change this comment in the duplicated frame to describe this message."
        n105 = Merge Errors(w241) -> (w237:errorcluster)
        n106 = call-poly "Enqueue Message.vi"("error in (no error)"=w237, "Message"="Tags Created", "Message Queue"=w236) -> ("error out"=w228:errorcluster)  [unwired: 7 in, 1 out]
        n107 = call "Generate Temporary Report.vi"("error in (no error)"=w228, "Line of Events"=string[] ["Create Tags Recieved"], "Module Name"=w229) -> ("error out"=w227:errorcluster)  [unwired: 8 in]
        n108 = Unbundle By Name(w232) -> ("Pump Module Config.Process Name"=w235:string)
        n109 = Concatenate Strings(w235, " Tags Made" ("text")) -> (w233:string)
        n110 = call "Write to Log File.vi"("error in"=w227, "text"=w233) -> ()  [unwired: 9 in, 1 out]
      }
      frame "Acquisition Stopped" {
        # "Logic for determining what action to take when the acquisition has stopped."
        n111 = case shown="\"Waiting for Stop (Log Stopped)\"" w251 {
          selector: w251 -> [w254 _ _ _ _]
          tunnel: [w254 UI_State."Waiting for Exit (Acq Stopped)" ("UI State") UI_State."Waiting for Stop (Acq Stopped)" ("UI State") UI_State."Idle" ("UI State") UI_State."Idle" ("UI State")] -> w250
          tunnel: w249 -> [w253 w255 w257 w263 w269]
          tunnel: [w253 w255 w257 w262 w268] -> w244
          tunnel: w248 -> [_ _ _ w261 w267]
          frame Default {
          }
          frame "Waiting for Exit", "Waiting for Exit (Acq Stopped)" {
          }
          frame "Waiting for Stop", "Waiting for Stop (Acq Stopped)" {
          }
          frame "Waiting for Exit (Log Stopped)" {
            # "If we are waiting to exit, and the logging has already stopped, then the \"Acquisition Stopped\" message indicates that it is time to exit."
            n112 = call-poly "Enqueue Message.vi"("Priority Message? (F)"=TRUE, "error in (no error)"=w263, "Message"="Exit", "Message Queue"=w261) -> ("error out"=w262:errorcluster)  [unwired: 6 in, 1 out]
          }
          frame "Waiting for Stop (Log Stopped)" {
            # "If we are waiting to stop, and the logging has already stopped, then the \"Acquisition Stopped\" message indicates that it is time to stop."
            n113 = call-poly "Enqueue Message.vi"("error in (no error)"=w269, "Message Data"="Ready..." ("Message"), "Message"="Update Status", "Message Queue"=w267) -> ("error out"=w268:errorcluster)  [unwired: 6 in, 1 out]
          }
        }
        n114 = Unbundle By Name(w243) -> ("Pump Module Config.Process Name"=w247:string)
        n115 = Concatenate Strings(w247, " Aquisition Stopped" ("text")) -> (w245:string)
        n116 = call "Write to Log File.vi"("error in"=w244, "text"=w245) -> ()  [unwired: 9 in, 1 out]
      }
      frame "Broadcast Settings" {
        # "Send the 'Update Settings' message to the Logging and Acquisition message loops."
        n117 = Unbundle By Name(w288) -> ("Pump Module Config"=w295:T3, "Pump Module Config.Settings.Cycle Period"=w285:dbl)
        n118 = call "Cycle Period FGV.vi"("Write"=TRUE, "error in (no error)"=w283, "Cycle Period In (ms)"=w285) -> ("error out"=w282:errorcluster)  [unwired: 7 in, 1 out]
        n119 = call "Broadcast Pump Settings.vi"("error in (no error)"=w282, "Message Queues"=w296, "Pump Module Config"=w295) -> ("error out"=w297:errorcluster)  [unwired: 8 in]
        n120 = Unbundle By Name(w295) -> ("Load Count"=w294:i32, "Settings.Output Device"=w291:T5)
        n121 = call-poly "Enqueue Message.vi"("error in (no error)"=w297, "Message Data"=w295, "Message"="Commit Config (Pump Module)", "Message Queue"=w298) -> ("error out"=w293:errorcluster)  [unwired: 6 in, 1 out]
        n122 = case "Is a device selected" shown="\"Ismatec ISM 831C\"..\"VICI M6\"" w291 {
          tunnel: w293 -> [w302 w306]
          tunnel: w292 -> [_ w305]
          tunnel: [w302 w304] -> w276
          tunnel: w294 -> [_ w303]
          frame "Default", Default {
          }
          frame "Ismatec ISM 831C".."VICI M6" {
            n123 = case "If it's first opened, put it in pause" shown="0" w303 {
              tunnel: w306 -> [w307 w311]
              tunnel: w305 -> [_ w310]
              tunnel: [w307 w314] -> w304
              frame Default {
              }
              frame 0 {
                n124 = call-poly "Enqueue Message.vi"("error in (no error)"=w311, "Message"="Start", "Message Queue"=w310) -> ("error out"=w308:errorcluster, "dup Message Queue"=w309:refnum<queue>)  [unwired: 7 in]
                n125 = call-poly "Enqueue Message.vi"("error in (no error)"=w308, "Message"="Pause", "Message Queue"=w309) -> ("error out"=w314:errorcluster)  [unwired: 7 in, 1 out]
              }
            }
          }
        }
        n126 = Unbundle By Name(w288) -> ("Pump Module Config.User name"=w271:string, "Pump Module Config.Process Name"=w274:string, "Pump Module Config.Settings"=w287:T4)
        n127 = Flatten To XML(anything=w287) -> (xml string=w272:string)
        n128 = Search and Replace String(replace all?=TRUE ("replace all? (F)"), input string=w272, search string="\r\n", replace string="_" ("replace string (\"\")")) -> (result string=w273:string)  [unwired: 4 in, 3 out]
        n129 = Build Array (concatenate)(string[] ["Settings Broadcast"] ("Line of Events"), w273) -> (w277:string[])
        n130 = call "Generate Temporary Report.vi"("error in (no error)"=w276, "Line of Events"=w277, "Module Name"=w274) -> ("error out"=w275:errorcluster)  [unwired: 8 in]
        n131 = Concatenate Strings(w274, " Broadcast Settings: " ("text"), w272) -> (w289:string)
        n132 = property class="VI"("Front Panel.Title"=w271) -> ()  [unwired: 2 in, 2 out]
        n133 = property on="User Name" class="Str"("Value"=w271) -> ()  [unwired: 2 in, 2 out]
        n134 = call "Write to Log File.vi"("error in"=w275, "text"=w289) -> ()  [unwired: 9 in, 1 out]
      }
      frame "Sequence Update" {
        n135 = in-place {
          in-place-border: w325 -> [w338]
          in-place-border: w323 -> [w337]
          in-place-border: [w336] -> w322
          n136 = in-place-cluster #1(w317) -> ("Pump Module Config"=w334:T3)
          n137 = Variant To Data(error in=w337, type=T26 {"Auto?"=TRUE, "Manual Entry"=0.0, "Setpoint"=0.0} ("Cluster"), Variant=w338) -> (data=w340:T26, error out=w336:errorcluster)
          n138 = Unbundle By Name(w340) -> ("Manual Entry"=w339:dbl)
          n139 = Bundle By Name(cluster=w334, "Settings.Manual Entry"=w339) -> (w335:T3)
          n140 = in-place-cluster #1("Pump Module Config"=w335) -> (w316:T19)
        }
        n141 = disable-structure shown="Disabled" {
          disable-tunnel: [w332 w333] -> w328
          disable-tunnel: w324 -> [w330 _]
          disable-tunnel: w322 -> [w329 w333]
          frame Disabled {
            n142 = call-poly "Enqueue Message.vi"("error in (no error)"=w329, "Message"="Broadcast Settings", "Message Queue"=w330) -> ("error out"=w332:errorcluster)  [unwired: 7 in, 1 out]
          }
          frame Enabled {
          }
        }
        n143 = Merge Errors(w328) -> (w319:errorcluster)
        n144 = Unbundle By Name(w316) -> ("Pump Module Config.Process Name"=w321:string)
        n145 = Concatenate Strings(w321, "Sequence Update" ("text")) -> (w318:string)
        n146 = call "Write to Log File.vi"("error in"=w319, "text"=w318) -> ()  [unwired: 9 in, 1 out]
      }
      frame "Send to Sequence Total" {
        n147 = Variant To Data(error in=w345, type=refnum<queue> refnum ("Message Queue"), Variant=w342) -> (data=w348:refnum<queue>, error out=w344:errorcluster)
        n148 = local read "Display Cluster"() -> (w347:T2)
        n149 = Unbundle By Name(w347) -> ("Total ml"=w346:dbl)
        n150 = call-poly "Enqueue Message.vi"("error in (no error)"=w344, "Message Data"=w346, "Message"="Sent to Sequence", "Message Queue"=w348) -> ("error out"=w343:errorcluster)  [unwired: 6 in, 1 out]
      }
      frame "Confirm Quit" {
        # "Confirm Quit - Message that can confirm whether or not the user wants to exit the application."
        n151 = case shown="\"Acquiring and Logging\"" w361 {
          tunnel: w360 -> [w367 w374]
          tunnel: w359 -> [w366 w372]
          tunnel: [w363 w371] -> w357
          tunnel: [UI_State."Idle" ("UI State") w370] -> w358
          tunnel: w356 -> [_ w369]
          frame Default {
            # "If 'Confirm Quit' comes in while the system is idle, there is no need for a confirmation message."
            n152 = call-poly "Enqueue Message.vi"("Priority Message? (F)"=TRUE, "error in (no error)"=w366, "Message"="Exit", "Message Queue"=w367) -> ("error out"=w363:errorcluster)  [unwired: 6 in, 1 out]
          }
          frame "Acquiring and Logging" {
            n153 = Two Button Dialog(message="Are you sure you want to quit while the acquisition is running?" ("Confirm Quit Message"), 1:"No" ("No"), 2:"Yes" ("Yes")) -> (T button?=w373:bool)
            n154 = case shown="True" w373 {
              tunnel: w374 -> [_ w388]
              tunnel: w372 -> [w378 w387]
              tunnel: [w378 w380] -> w371
              tunnel: [UI_State."Acquiring and Logging" ("UI State") UI_State."Waiting for Exit" ("UI State")] -> w370
              tunnel: w369 -> [_ w381]
              frame False {
                # "User did not want to quit."
              }
              frame True {
                n155 = call-poly "Enqueue Message.vi"("error in (no error)"=w387, "Message"="Stop", "Message Queue"=w388) -> ("error out"=w380:errorcluster)  [unwired: 7 in, 1 out]
                n156 = Unbundle By Name(w381) -> ("Pump Module Config.Process Name"=w383:string)
                n157 = Concatenate Strings(w383, " Quit" ("text")) -> (w384:string)
                n158 = call "Write to Log File.vi"("error in"=w380, "text"=w384) -> ()  [unwired: 9 in, 1 out]
              }
            }
          }
        }
      }
      frame "Display Log File Path" {
        n159 = Variant To Data(error in=w392, type=path "", Variant=w395) -> (data=→"Log File path":path, error out=w393:errorcluster)
      }
      frame "E-Stop" {
        # "Pause the pump when there is an E-STOP"
        # "Message Acquisition and Logging loops to stop"
        # "Enable: Start, Exit, Settings\nDisable: Stop"
        # "Stop the pumps."
        n160 = Unbundle By Name(w424) -> ("Trigger Ref"=w415:refnum<vi>, "Stop Ref"=w416:refnum<vi>, "Start Ref"=w419:refnum<vi>, "Exit Ref"=w418:refnum<vi>, "Settings Ref"=w417:refnum<vi>)
        n161 = call-poly "Enqueue Message.vi"("error in (no error)"=w408, "Message Data"="Ready..." ("Ready..."), "Message"="Update Status", "Message Queue"=w427) -> ("error out"=w410:errorcluster)  [unwired: 6 in, 1 out]
        n162 = Build Array(w419, w418, w417) -> (w422:refnum<vi>[])
        n163 = Build Array(w415, w416) -> (w421:refnum<vi>[])
        n164 = call-poly "Enqueue Message.vi"("error in (no error)"=w410, "Message"="Pause", "Message Queue"=w412) -> ("error out"=w409:errorcluster)  [unwired: 7 in, 1 out]
        n165 = call "Set Enable State on Multiple Controls.vi"("Enable?"=FALSE, "Controls"=w421) -> ()  [unwired: 10 in]
        n166 = call "Set Enable State on Multiple Controls.vi"("Enable?"=TRUE, "Controls"=w422) -> ()  [unwired: 10 in]
        n167 = case shown="Default" w413 {
          selector: w413 -> [_ w429]
          tunnel: [UI_State."Waiting for Stop" ("UI State") w429] -> w414
          frame Default {
          }
          frame "Waiting for Exit" {
          }
        }
        n168 = Merge Errors(w409) -> (w400:errorcluster)
        n169 = Bundle By Name(cluster=w406, "State"=State_Enum."Idle") -> (w403:T19)
        n170 = Unbundle By Name(w403) -> ("Pump Module Config.Process Name"=w398:string)
        n171 = call "Generate Temporary Report.vi"("error in (no error)"=w400, "Line of Events"=string[] ["E-STOP Recieved"], "Module Name"=w398) -> ("error out"=w399:errorcluster)  [unwired: 8 in]
        n172 = Concatenate Strings(w398, " E-STOP" ("text")) -> (w404:string)
        n173 = call "Write to Log File.vi"("error in"=w399, "text"=w404) -> ()  [unwired: 9 in, 1 out]
      }
      frame "Error" {
        # "Error - Check the error message data and respond accordingly. This message is sent by the \"Error Handler\" VIs at the end of each loop in this application."
        n174 = Variant To Data(error in=w446, type=errorcluster {"status"=FALSE, "code"=0, "source"=""} ("error out"), Variant=w445) -> (data=w443:errorcluster, error out=w439:errorcluster)
        n175 = call <vilib>:"General Error Handler.vi"("error in (no error)"=w443) -> ("message"=w432:string)  [unwired: 10 in, 4 out]
        n176 = call-poly "Enqueue Message.vi"("Priority Message? (F)"=TRUE, "Message"="Exit", "Message Queue"=w442) -> ("error out"=w438:errorcluster)  [unwired: 7 in, 1 out]
        n177 = Merge Errors(w438, w439) -> (w431:errorcluster)
        n178 = Unbundle By Name(w433) -> ("Pump Module Config.Process Name"=w436:string)
        n179 = Concatenate Strings(w436, " Error: " ("text"), w432) -> (w434:string)
        n180 = call "Write to Log File.vi"("error in"=w431, "text"=w434) -> ()  [unwired: 9 in, 1 out]
      }
      frame "Exit" {
        w464 = TRUE  # Delete Module?
        # "Don't check the error outs. The acquisition and logging queues may have already been released."
        # "Close references owned by the Main VI."
        # "Stop the VI"
        # "Exit - Fire the User Event to stop the Event Handling Loop.  Also send Exit messages to the Acquisition and Logging loops."
        n181 = Release Queue(queue=w472, error in (no error)=w476) -> (error out=w470:errorcluster)  [unwired: 1 in, 2 out]
        n182 = call "Fire User Event - Stop.vi"("User Event - Stop"=w475) -> ("error out"=w474:errorcluster)  [unwired: 10 in]
        n183 = Release Notifier(notifier=w471, error in (no error)=w470) -> (error out=w469:errorcluster)  [unwired: 1 in, 2 out]
        n184 = Release Queue(queue=w467, error in (no error)=w469) -> (error out=w468:errorcluster)  [unwired: 1 in, 2 out]
        n185 = call-poly "Enqueue Message.vi"("Message"="Stop", "Message Queue"=w459) -> ("dup Message Queue"=w457:refnum<queue>)  [unwired: 8 in, 1 out]
        n186 = Variant To Data(type=w464, Variant=w460) -> (data=w463:bool, error out=w465:errorcluster)  [unwired: 1 in]
        n187 = Select(t=w464, s=w465, f=w463) -> (s? t:f=w462:bool)
        n188 = call-poly "Enqueue Message.vi"("Message"="Exit", "Message Queue"=w457) -> ()  [unwired: 8 in, 2 out]
        n189 = case "Don't enqueue Delete Module if opening campaign because it\nwill already have been deleted and new config loaded and we create\na race condition." shown="True" w462 {
          tunnel: w461 -> [_ w480]
          tunnel: w453 -> [_ w479]
          frame False {
          }
          frame True {
            n190 = Unbundle By Name(w479) -> ("Pump Module Config.GUID"=w478:string)
            n191 = call-poly "Enqueue Message.vi"("Message Data"=w478, "Message"="Delete Module", "Message Queue"=w480) -> ()  [unwired: 7 in, 2 out]
          }
        }
        n192 = Merge Errors(w474, w468) -> (w449:errorcluster)
        n193 = Unbundle By Name(w453) -> ("Pump Module Config.Process Name"=w450:string)
        n194 = Concatenate Strings(w450, " Exit" ("text")) -> (w454:string)
        n195 = call "Generate Temporary Report.vi"("error in (no error)"=w449, "Line of Events"=string[] ["Exited"], "Module Name"=w450) -> ("error out"=w448:errorcluster)  [unwired: 8 in]
        n196 = call "Write to Log File.vi"("error in"=w448, "text"=w454) -> ()  [unwired: 9 in, 1 out]
      }
      frame "Init UI Refs" {
        # "Enable: Start, Exit, Settings\nDisable: Stop"
        # "Init UI Refs - Store control references for UI controls.  Also enable/disable controls appropriately."
        n197 = property class="VI"("Front Panel.Closeable"=TRUE ("Front Panel Window:Closeable")) -> ()  [unwired: 2 in, 2 out]
        n198 = control-ref of="Status"() -> (w488:refnum<vi>)
        n199 = control-ref of="Exit"() -> (w485:refnum<vi>)
        n200 = Bundle By Name(cluster=w491, "Status Ref"=w488, "Exit Ref"=w485) -> (w490:T18)
        n201 = Build Array(w485) -> (w487:refnum<vi>[])
        n202 = call "Set Enable State on Multiple Controls.vi"("Enable?"=TRUE, "Controls"=w487) -> ()  [unwired: 10 in]
      }
      frame "Initialize" {
        # "Initialize - Get configuration settings, then message the UI to initialize, and broadcast the settings to the other message loops."
        n203 = property class="VI" props=["FP.State"]() -> (reference out=w504:refnum<vi>)  [unwired: 2 in, 2 out]
        n204 = call-poly "Enqueue Message.vi"("error in (no error)"=w505, "Message"="Init UI Refs", "Message Queue"=w510) -> ("error out"=w508:errorcluster, "dup Message Queue"=w509:refnum<queue>)  [unwired: 7 in]
        n205 = call "Make Child and Move.vi"("Process Name"=w501, "Name of Parent Panel"=w502, "New Center Coords"=w503, "VI in"=w504) -> ()  [unwired: 8 in]
        n206 = call-poly "Enqueue Message.vi"("error in (no error)"=w508, "Message"="Broadcast Settings", "Message Queue"=w509) -> ("error out"=w516:errorcluster, "dup Message Queue"=w515:refnum<queue>)  [unwired: 7 in]
        n207 = call-poly "Enqueue Message.vi"("error in (no error)"=w516, "Message Data"="Ready..." ("Ready..."), "Message"="Update Status", "Message Queue"=w515) -> ("error out"=w494:errorcluster)  [unwired: 6 in, 1 out]
        n208 = Unbundle By Name(w498) -> ("Pump Module Config.Process Name"=w495:string)
        n209 = call "Generate Temporary Report.vi"("error in (no error)"=w494, "Line of Events"=string[] ["Initialized"], "Module Name"=w495) -> ("error out"=w493:errorcluster)  [unwired: 8 in]
        n210 = Concatenate Strings(w495, " Initialize" ("text")) -> (w499:string)
        n211 = call "Write to Log File.vi"("error in"=w493, "text"=w499) -> ()  [unwired: 9 in, 1 out]
      }
      frame "Launch Settings Dialog" {
        # "Keep track of the number of times it has opened"
        # "Launch the Settings Dialog when the user clicks the 'Settings' button."
        n212 = in-place {
          n213 = in-place-cluster #2(w523) -> ("Pump Module Config.Load Count"=w560:i32)
          n214 = Increment(x=w560) -> (x+1=w559:i32)
          n215 = in-place-cluster #2("Pump Module Config.Load Count"=w559) -> (w519:T19)
        }
        n216 = call-by-ref "?"("error in (no error)"=w533, "Message Queues"=w532, "Pump Module State Cluster In"=w519) -> ("error out"=w530:errorcluster, "Cancelled?"=w529:bool, "Pump Module Config Out"=w531:T3)  [unwired: 7 in, 3 out]
        n217 = Unbundle By Name(w519) -> ("Pump Module Config.Settings.Output Device"=w518:T5)
        n218 = case shown="True" w529 {
          tunnel: [w561 w565] -> w524
          tunnel: w534 -> [_ w564]
          tunnel: w530 -> [w561 w562]
          frame False {
          }
          frame True {
            # "Send out the settings"
            n219 = call-poly "Enqueue Message.vi"("error in (no error)"=w562, "Message"="Broadcast Settings", "Message Queue"=w564) -> ("error out"=w565:errorcluster)  [unwired: 7 in, 1 out]
          }
        }
        n220 = Bundle By Name(cluster=w523, "Pump Module Config"=w531) -> (w525:T19)
        n221 = Unbundle By Name(w525) -> ("Pump Module Config.Settings.Pump Cal Enum"=→"Calibration Enum":u16, "Pump Module Config.Process Name"=w528:string, "Pump Module Config.Settings.Output Device"=w520:T5)
        n222 = Equal?(x=w520, y=w518) -> (x = y?=w517:bool)
        n223 = case shown="False" w517 {
          tunnel: w520 -> [w537 _]
          frame False {
            n224 = control-ref of="This VI"() -> (w543:refnum<vi>)
            n225 = property class="VI"(reference=w543) -> (reference out=w538:refnum<vi>, "Front Panel.PanelBounds"=w542:T24)  [unwired: 1 in, 1 out]
            n226 = Unbundle By Name(w542) -> ("Bottom"=w540:i16)
            n227 = case shown="\"Masterflex 75211-70\"" w537 {
              tunnel: w540 -> [w545 w549 w551]
              tunnel: [w544 w548 w550] -> w539
              frame "Default", Default {
                n228 = Subtract(x=w545, y=i16 35) -> (x-y=w544:i16)
              }
              frame "SSI PR/LD", "SSI P40" {
                n229 = Add(x=w549, y=i16 23) -> (x+y=w548:i16)
              }
              frame "Masterflex 75211-70" {
                n230 = Add(x=w551, y=i16 35) -> (x+y=w550:i16)
              }
            }
            n231 = Bundle By Name(cluster=w542, "Bottom"=w539) -> (w541:T24)
            n232 = property class="VI"(reference=w538, "Front Panel.PanelBounds"=w541) -> ()  [unwired: 1 in, 2 out]
          }
          frame True {
          }
        }
        n233 = case shown="\"ASIA Type C\"" w520 {
          frame "Default", Default {
            n234 = call <userlib>:"Current VI's Path__ogtk.vi"() -> ("Current VI's Path (+ Relative)"=w555:path)  [unwired: 1 in]
            n235 = Open VI Reference(vi path=w555) -> (vi reference=w554:refnum<vi>)  [unwired: 5 in, 1 out]
            n236 = property class="VI"(reference=w554, "Front Panel.ShowMenuBar"=FALSE ("Front Panel Window:Show Menu Bar")) -> ()  [unwired: 1 in, 2 out]
          }
          frame "ASIA Type C" {
            n237 = call <userlib>:"Current VI's Path__ogtk.vi"() -> ("Current VI's Path (+ Relative)"=w558:path)  [unwired: 1 in]
            n238 = Open VI Reference(vi path=w558) -> (vi reference=w557:refnum<vi>)  [unwired: 5 in, 1 out]
            n239 = property class="VI"(reference=w557, "Front Panel.ShowMenuBar"=TRUE ("Front Panel Window:Show Menu Bar")) -> ()  [unwired: 1 in, 2 out]
          }
        }
        n240 = Concatenate Strings(w528, " Setting Dialog Launched" ("text")) -> (w526:string)
        n241 = call "Write to Log File.vi"("error in"=w524, "text"=w526) -> ()  [unwired: 9 in, 1 out]
      }
      frame "Logging Stopped" {
        # "Logic for determining what action to take when the logging has stopped."
        n242 = case shown="\"Waiting for Exit (Acq Stopped)\"" w575 {
          selector: w575 -> [w578 _ _ _ _]
          tunnel: [w578 UI_State."Waiting for Exit (Log Stopped)" ("UI State") UI_State."Waiting for Stop (Log Stopped)" ("UI State") UI_State."Idle" ("UI State") UI_State."Idle" ("UI State")] -> w574
          tunnel: w573 -> [w577 w579 w581 w587 w593]
          tunnel: [w577 w579 w581 w586 w592] -> w567
          tunnel: w572 -> [_ _ _ w585 w591]
          frame Default {
          }
          frame "Waiting for Exit", "Waiting for Exit (Log Stopped)" {
          }
          frame "Waiting for Stop", "Waiting for Stop (Log Stopped)" {
          }
          frame "Waiting for Exit (Acq Stopped)" {
            # "If we are waiting to exit, and the acquisition has already stopped, then the \"Logging Stopped\" message indicates that it is time to exit."
            n243 = call-poly "Enqueue Message.vi"("Priority Message? (F)"=TRUE, "error in (no error)"=w587, "Message"="Exit", "Message Queue"=w585) -> ("error out"=w586:errorcluster)  [unwired: 6 in, 1 out]
          }
          frame "Waiting for Stop (Acq Stopped)" {
            # "If we are waiting to stop, and the acquisition has already stopped, then the \"Logging Stopped\" message indicates that it is time to stop."
            n244 = call-poly "Enqueue Message.vi"("error in (no error)"=w593, "Message Data"="Ready..." ("Message"), "Message"="Update Status", "Message Queue"=w591) -> ("error out"=w592:errorcluster)  [unwired: 6 in, 1 out]
          }
        }
        n245 = Unbundle By Name(w568) -> ("Pump Module Config.Process Name"=w571:string)
        n246 = Concatenate Strings(w571, " Logging Stopped" ("text")) -> (w569:string)
        n247 = call "Write to Log File.vi"("error in"=w567, "text"=w569) -> ()  [unwired: 9 in, 1 out]
      }
      frame "Start" {
        # "Clear chart"
        # "Message Acquisition and Logging loops to start"
        # "Enable: Stop\nDisable: Start, Exit, Settings"
        # "Start - Enable/Disable buttons appropriately for an acquisition that has started, and update status display."
        n248 = Unbundle By Name(w603) -> ("Trigger Ref"=w611:refnum<vi>, "Stop Ref"=w612:refnum<vi>, "Start Ref"=w615:refnum<vi>, "Exit Ref"=w614:refnum<vi>, "Settings Ref"=w613:refnum<vi>, "Data Ref"=w605:refnum<vi>)
        n249 = property class="WFChart (strict)"(reference=w605, "History Data"=waveform(dbl)[][] []) -> ()  [unwired: 1 in, 2 out]
        n250 = Build Array(w615, w614, w613) -> (w618:refnum<vi>[])
        n251 = Build Array(w611, w612) -> (w617:refnum<vi>[])
        n252 = call "Set Enable State on Multiple Controls.vi"("Enable?"=TRUE, "Controls"=w617) -> ()  [unwired: 10 in]
        n253 = call "Set Enable State on Multiple Controls.vi"("Enable?"=FALSE, "Controls"=w618) -> ()  [unwired: 10 in]
        n254 = call-poly "Enqueue Message.vi"("error in (no error)"=w606, "Message"="Broadcast settings", "Message Queue"=w608) -> ("error out"=w609:errorcluster, "dup Message Queue"=w607:refnum<queue>)  [unwired: 7 in]
        n255 = in-place {
          in-place-border: w609 -> [w624]
          in-place-border: w607 -> [w623]
          in-place-border: [w622] -> w595
          n256 = in-place-cluster #3(w599) -> ("State"=w621:T20)
          n257 = case shown="Default" w621 {
            tunnel: [w626 w629] -> w625
            tunnel: w624 -> [w626 w628]
            tunnel: w623 -> [_ w627]
            frame "Measuring" {
            }
            frame Default {
              # "If it is not started yet, start"
              n258 = call-poly "Enqueue Message.vi"("error in (no error)"=w628, "Message"="Start Loops", "Message Queue"=w627) -> ("error out"=w629:errorcluster)  [unwired: 7 in, 1 out]
            }
          }
          n259 = in-place-cluster #3("State"=State_Enum."Measuring") -> (w598:T19)
          n260 = Merge Errors(w625) -> (w622:errorcluster)
        }
        n261 = Unbundle By Name(w598) -> ("Pump Module Config.Process Name"=w596:string)
        n262 = Concatenate Strings(w596, " Start" ("text")) -> (w601:string)
        n263 = call "Write to Log File.vi"("error in"=w595, "text"=w601) -> ()  [unwired: 9 in, 1 out]
      }
      frame "Sequence Start" {
        # "Clear chart"
        # "Message Acquisition and Logging loops to start"
        # "Enable: Stop\nDisable: Start, Exit, Settings"
        # "Start - Enable/Disable buttons appropriately for an acquisition that has started, and update status display."
        n264 = Unbundle By Name(w643) -> ("Trigger Ref"=w650:refnum<vi>, "Stop Ref"=w651:refnum<vi>, "Start Ref"=w654:refnum<vi>, "Exit Ref"=w653:refnum<vi>, "Settings Ref"=w652:refnum<vi>, "Data Ref"=w645:refnum<vi>)
        n265 = property class="WFChart (strict)"(reference=w645, "History Data"=waveform(dbl)[][] []) -> ()  [unwired: 1 in, 2 out]
        n266 = Build Array(w654, w653, w652) -> (w657:refnum<vi>[])
        n267 = Build Array(w650, w651) -> (w656:refnum<vi>[])
        n268 = call-poly "Enqueue Message.vi"("error in (no error)"=w646, "Message"="Broadcast settings", "Message Queue"=w647) -> ("error out"=w631:errorcluster, "dup Message Queue"=w632:refnum<queue>)  [unwired: 7 in]
        n269 = call "Set Enable State on Multiple Controls.vi"("Enable?"=TRUE, "Controls"=w656) -> ()  [unwired: 10 in]
        n270 = call "Set Enable State on Multiple Controls.vi"("Enable?"=FALSE, "Controls"=w657) -> ()  [unwired: 10 in]
        n271 = case shown="False" w638 {
          selector: w638 -> [_ w664]
          tunnel: [TRUE w664] -> w640
          tunnel: w631 -> [w662 w665]
          tunnel: w632 -> [w660 _]
          tunnel: [w659 w665] -> w639
          frame False {
            # "Start the loop if it isn't started yet"
            n272 = call-poly "Enqueue Message.vi"("error in (no error)"=w662, "Message"="Start Loops", "Message Queue"=w660) -> ("error out"=w659:errorcluster)  [unwired: 7 in, 1 out]
          }
          frame True {
          }
        }
        n273 = Bundle By Name(cluster=w642, "State"=State_Enum."Measuring") -> (w633:T19)
        n274 = Merge Errors(w639) -> (w634:errorcluster)
        n275 = Unbundle By Name(w633) -> ("Pump Module Config.Process Name"=w637:string)
        n276 = Concatenate Strings(w637, " Sequence Start" ("text")) -> (w635:string)
        n277 = call "Write to Log File.vi"("error in"=w634, "text"=w635) -> ()  [unwired: 9 in, 1 out]
      }
      frame "Start Loops" {
        # "I don't think we would have multiple loops but i'm leaving it here incase."
        # "Message Acquisition and Logging loops to start"
        # "Start - Enable/Disable buttons appropriately for an acquisition that has started, and update status display."
        n278 = Unbundle By Name(w672) -> ("Pump Module Config.Process Name"=w668:string)
        n279 = Build Array(w675) -> (w673:refnum<queue>[])
        n280 = for {
          tunnel: w671 -> [w681]
          tunnel: [w680] -> w674 mode=indexing
          tunnel: w673 -> [w679] mode=indexing
          tunnel: w668 -> [w678]
          n281 = call-poly "Enqueue Message.vi"("error in (no error)"=w681, "Message Data"=w678, "Message"="Start", "Message Queue"=w679) -> ("error out"=w680:errorcluster)  [unwired: 6 in, 1 out]
        }
        n282 = Merge Errors(w671, w674) -> (w667:errorcluster)
        n283 = call "Generate Temporary Report.vi"("error in (no error)"=w667, "Line of Events"=string[] ["Started"], "Module Name"=w668) -> ("error out"=w666:errorcluster)  [unwired: 8 in]
      }
      frame "Start Log" {
        # "Message Acquisition and Logging loops to start"
        # "Start - Enable/Disable buttons appropriately for an acquisition that has started, and update status display."
        n284 = Unbundle By Name(w685) -> ("Pump Module Config.Process Name"=w690:string)
        n285 = Build Array(w693) -> (w691:refnum<queue>[])
        n286 = for {
          tunnel: w684 -> [w699]
          tunnel: [w698] -> w692 mode=indexing
          tunnel: w691 -> [w697] mode=indexing
          tunnel: w690 -> [w696]
          n287 = call-poly "Enqueue Message.vi"("error in (no error)"=w699, "Message Data"=w696, "Message"="Start Log", "Message Queue"=w697) -> ("error out"=w698:errorcluster)  [unwired: 6 in, 1 out]
        }
        n288 = Merge Errors(w684, w692) -> (w686:errorcluster)
        n289 = Unbundle By Name(w685) -> ("Pump Module Config.Process Name"=w689:string)
        n290 = Concatenate Strings(w689, " Start Log" ("text")) -> (w687:string)
        n291 = call "Write to Log File.vi"("error in"=w686, "text"=w687) -> ()  [unwired: 9 in, 1 out]
      }
      frame "Stop" {
        # "Pause the pump when we get a stop command"
        # "Enable: Start, Exit, Settings\nDisable: Stop"
        # "Stop - Enable/Disable buttons appropriately for an acquisition that has stopped, and update status display."
        n292 = Unbundle By Name(w731) -> ("Trigger Ref"=w722:refnum<vi>, "Stop Ref"=w723:refnum<vi>, "Start Ref"=w726:refnum<vi>, "Exit Ref"=w725:refnum<vi>, "Settings Ref"=w724:refnum<vi>)
        n293 = call-poly "Enqueue Message.vi"("error in (no error)"=w713, "Message"="Broadcast settings", "Message Queue"=w711) -> ("error out"=w712:errorcluster, "dup Message Queue"=w710:refnum<queue>)  [unwired: 7 in]
        n294 = Build Array(w726, w725, w724) -> (w729:refnum<vi>[])
        n295 = Build Array(w722, w723) -> (w728:refnum<vi>[])
        n296 = call-poly "Enqueue Message.vi"("error in (no error)"=w712, "Message Data"="Ready..." ("Ready..."), "Message"="Update Status", "Message Queue"=w710) -> ("error out"=w718:errorcluster)  [unwired: 6 in, 1 out]
        n297 = call "Set Enable State on Multiple Controls.vi"("Enable?"=FALSE, "Controls"=w728) -> ()  [unwired: 10 in]
        n298 = call "Set Enable State on Multiple Controls.vi"("Enable?"=TRUE, "Controls"=w729) -> ()  [unwired: 10 in]
        n299 = call-poly "Enqueue Message.vi"("error in (no error)"=w718, "Message"="Pause", "Message Queue"=w719) -> ("error out"=w716:errorcluster)  [unwired: 7 in, 1 out]
        n300 = case shown="Default" w720 {
          selector: w720 -> [_ w735]
          tunnel: [UI_State."Waiting for Stop" ("UI State") w735] -> w721
          frame Default {
          }
          frame "Waiting for Exit" {
          }
        }
        n301 = Merge Errors(w716) -> (w703:errorcluster)
        n302 = Bundle By Name(cluster=w715, "State"=State_Enum."Paused") -> (w706:T19)
        n303 = Unbundle By Name(w706) -> ("Pump Module Config.Process Name"=w701:string)
        n304 = call "Generate Temporary Report.vi"("error in (no error)"=w703, "Line of Events"=string[] ["Stopped"], "Module Name"=w701) -> ("error out"=w702:errorcluster)  [unwired: 8 in]
        n305 = Concatenate Strings(w701, " Stop" ("text")) -> (w707:string)
        n306 = call "Write to Log File.vi"("error in"=w702, "text"=w707) -> ()  [unwired: 9 in, 1 out]
      }
      frame "Update Status" {
        # "Update Display - Convert the message data to a string to display in the Status indicator."
        n307 = Variant To Data(error in=w747, type="", Variant=w746) -> (data=w740:string, error out=w744:errorcluster)
        "Status" <- w740
        n308 = Unbundle By Name(w743) -> ("Trigger Ref"=w739:refnum<vi>, "Stop Ref"=w742:refnum<vi>)
        n309 = property class="Bool"(reference=w742) -> ("DisabledEnum"=w741:T27)  [unwired: 1 in, 2 out]
        n310 = case shown="\"Enabled\"" w741 {
          tunnel: w740 -> [w751 _]
          tunnel: w739 -> [w752 _]
          frame "Enabled" {
            # "Disable the Force Trigger only while we are logging."
            n311 = Build Array(w752) -> (w753:refnum<vi>[])
            n312 = Not Equal?(x="Logging" ("Logging"), y=w751) -> (x != y?=w749:bool)
            n313 = call "Set Enable State on Multiple Controls.vi"("Enable?"=w749, "Controls"=w753) -> ()  [unwired: 10 in]
          }
          frame "Disabled", Default {
          }
        }
        n314 = Merge Errors(w744) -> (w748:errorcluster)
      }
      frame "Empty ASIA", "Fill ASIA" {
        n315 = Unbundle By Name(w756) -> ("Pump Module Config.Settings.Output Device"=w755:T5)
        n316 = case shown="\"ASIA Type C\"" w755 {
          tunnel: w759 -> [_ w767]
          tunnel: w758 -> [w763 w766]
          tunnel: [w763 w765] -> w757
          tunnel: w754 -> [_ w764]
          frame "Default", Default {
          }
          frame "ASIA Type C" {
            n317 = call-poly "Enqueue Message.vi"("error in (no error)"=w766, "Message"=w764, "Message Queue"=w767) -> ("error out"=w765:errorcluster)  [unwired: 7 in, 1 out]
          }
        }
      }
      frame Default {
        # "'Default' case only runs if there is a message that isn't defined in any of the other cases.  Output a programming error."
        n318 = Concatenate Strings("The invalid message string " ("string"), w770, " was received in Pump Module Main." ("string")) -> (w771:string)
        n319 = Bundle By Name(cluster=errorcluster {"status"=TRUE, "code"=1, "source"=""} ("error constant"), "source"=w771) -> (w769:errorcluster)
        n320 = Unbundle By Name(w775) -> ("Pump Module Config.Process Name"=w778:string)
        n321 = Concatenate Strings(w778, " Incorrect Message Recieved: " ("text"), w770) -> (w776:string)
        n322 = call "Write to Log File.vi"("error in"=w769, "text"=w776) -> ()  [unwired: 9 in, 1 out]
      }
    }
    n323 = call "Error Handler - Message Handling Loop.vi"("error in (no error)"=w210, "Message Queue"=w208) -> ("dup error in"=w209:errorcluster, "dup Message Queue"=w194:refnum<queue>)  [unwired: 8 in]
  }
  "Sequence Started" <- w7
  n324 = call "Main Loop.vi"("error in (no error)"=w10, "Chart Notifier"=w17, "Message Queues"=w11) -> ("error out"=w18:errorcluster)  [unwired: 8 in]
  n325 = Release Queue(queue=w2) -> ()  [unwired: 2 in, 3 out]
  n326 = Close Reference(reference=w16) -> ()  [unwired: 1 in, 1 out]
  n327 = Unregister For Events(event registration refnum=w24, error in=w29) -> (error out=w25:errorcluster)
  n328 = Release Queue(queue=w4) -> ()  [unwired: 2 in, 3 out]
  n329 = Release Queue(queue=w3) -> ()  [unwired: 2 in, 3 out]
  n330 = Merge Errors(w25, w30, w10, w18) -> (w28:errorcluster)
  n331 = call "Destroy User Event - Stop.vi"("error in (no error)"=w28, "User Event - Stop"=w26) -> ()  [unwired: 9 in, 1 out]
